vi "Close Instrument Sessions.vi"(0 "SG Path Group in":refnum<class "SG Path Group.lvclass">, 11 "error in":errorcluster) -> (4 "SG Path Group out":refnum<class "SG Path Group.lvclass">, 15 "error out":errorcluster)   [LabVIEW 2023, in "RFFixtureCharact.PXI.lvlib" / "SG Path Group.lvclass"]
uses:
  SG Path Group.lvclass
  SG Path Group.lvclass/SG Path Group.ctl
  Instruments/Power Meter/Power Meter Factory/Power Meter Factory.lvclass
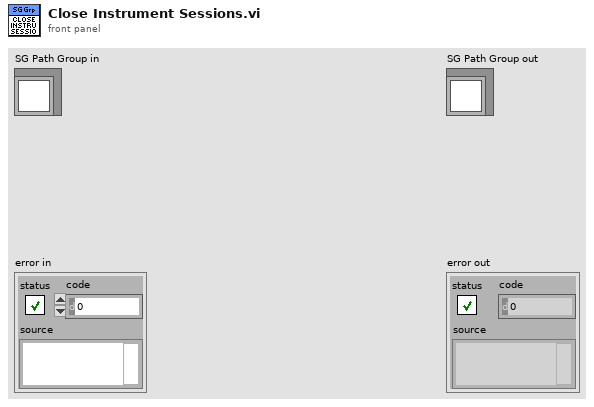
[diagram p1: front panel]
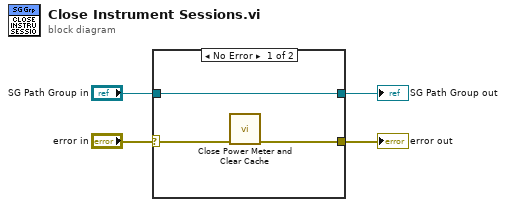
[diagram p0: block diagram]
diagram:
  n1 = case shown="No Error" "error in" {
    selector: "error in" -> [w6 w9]
    tunnel: [w7 w9] -> w1
    tunnel: [w5 w8] -> w2
    tunnel: "SG Path Group in" -> [w5 w8]
    frame No Error {
      n2 = call "Close Power Meter and Clear Cache.vi"("error in (no error)"=w6) -> ("error out"=w7:errorcluster)  [unwired: 14 in]
    }
    frame Error {
    }
  }
  "error out" <- w1
  "SG Path Group out" <- w2
